vi "Initialize MenuButton Event Handler.vi"(10 "Defer Panel Updates?(T)":bool=TRUE, 11 "Menu Buttons":refnum<class "MenuButton.lvclass">[](array[class])) -> (0 "error out":errorcluster, 3 "MenuButton Event Handler out":refnum<class "MenuButton Event Handler.lvclass">)   [LabVIEW 2017, in "MenuButtons.lvlib" / "MenuButton Event Handler.lvclass"]
uses:
  MenuButton Event Handler.lvclass
  MenuButton/MenuButton.lvclass
  MenuButton Event Handler.lvclass/MenuButton Event Handler.ctl
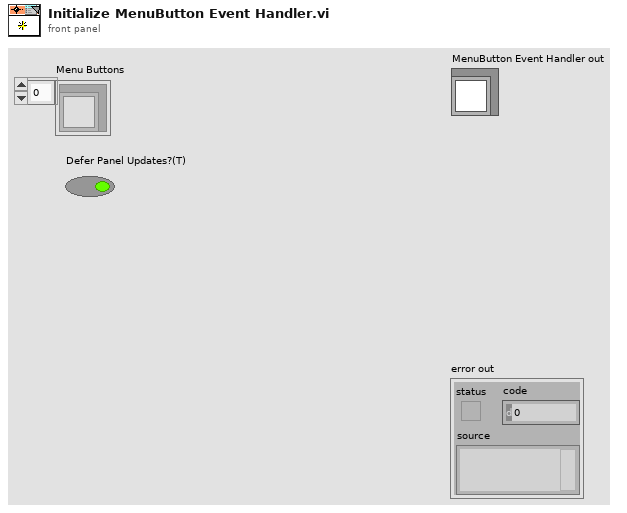
[diagram p1: front panel]
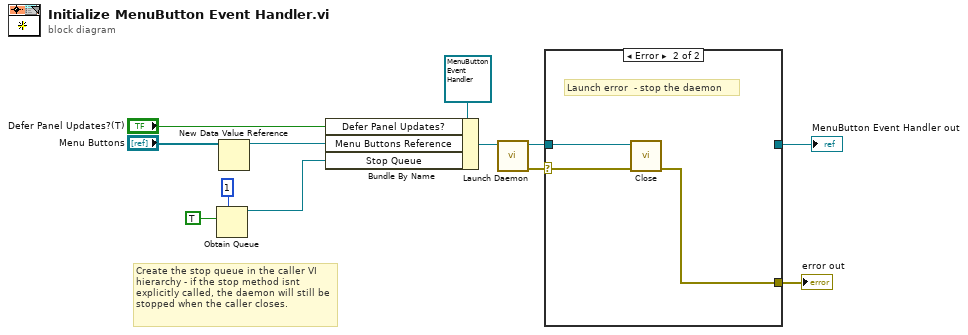
[diagram p0: block diagram]
diagram:
  # "Create the stop queue in the caller VI hierarchy - if the stop method isnt explicitly called, the daemon will still be stopped when the caller closes."
  n1 = Obtain Queue(max queue size (-1, unlimited)=1, element data type=TRUE) -> (queue out=w5:refnum<queue>)  [unwired: 3 in, 2 out]
  n2 = New Data Value Reference(data value="Menu Buttons") -> (data value reference=w11:refnum<data-value>)  [unwired: 1 in, 1 out]
  n3 = Bundle By Name(cluster=refnum<class "MenuButton Event Handler.lvclass"> refnum ("MenuButton Event Handler in"), "Defer Panel Updates?"="Defer Panel Updates?(T)", "Menu Buttons Reference"=w11, "Stop Queue"=w5) -> (w8:refnum<class "MenuButton Event Handler.lvclass">)
  n4 = call "Launch Daemon.vi"("MenuButton Event Handler in"=w8) -> ("error out"=w4:errorcluster, "MenuButton Event Handler out"=w3:refnum<class "MenuButton Event Handler.lvclass">)  [unwired: 9 in]
  n5 = case shown="Error" w4 {
    selector: w4 -> [w13 w16]
    tunnel: w3 -> [w14 w17]
    tunnel: [w14 _] -> w2
    tunnel: [w13 w15] -> w1
    frame No Error {
    }
    frame Error {
      # "Launch error  - stop the daemon"
      n6 = call "Close.vi"("error in (no error)"=w16, "MenuButton Event Handler in"=w17) -> ("error out"=w15:errorcluster)  [unwired: 9 in]
    }
  }
  "error out" <- w1
  "MenuButton Event Handler out" <- w2
